vi "Parse.vi"(8 "Error In":errorcluster, 11 "Reader":refnum<class "Abstract.lvclass">) -> (0 "Error Out":errorcluster, 3 "Tokens":refnum<class "Abstract.lvclass">[](array[class]))   [LabVIEW 2018, in "Toolkit.lvlib" / "Parser.lvclass"]
uses:
  Parser.lvclass
  Tokens/Abstract/Abstract.lvclass
  Readers/Abstract/Abstract.lvclass
  Parser.lvclass/Parser.ctl
  Support/Is Open Delimiter.vi
  Support/Pop Content.vi
  Support/Has Content.vi
  Support/Add Text Token.vi
  Support/Peek Content.vi
  Support/Is Close Delimiter.vi
  Support/Tokenize Tag.vi
  Support/Ignore Comment.vi
  Support/Change Delimiters.vi
  Tokens/Text/Text.lvclass
  D:/Users/cfield/Code/Field R&D Services/Mustache/trunk/src/Toolkit/Tokens/Abstract/Abstract.lvclass
  Tokens/EscapedVariable/EscapedVariable.lvclass
  D:/Users/cfield/Code/Field R&D Services/Mustache/trunk/src/Toolkit/Tokens/Keyable/API/Keyable.lvclass
  Tokens/UnescapedVariable/UnescapedVariable.lvclass
  Tokens/BeginSection/BeginSection.lvclass
  Tokens/InvertedSection/InvertedSection.lvclass
  Tokens/EndSection/EndSection.lvclass
  Tokens/Partial/Partial.lvclass
  Tokens/Keyable/API/Keyable.lvclass
  Tokens/Text/API/New.vi
  <vilib>/Utility/error.llb/Trim Whitespace.vi
  Tokens/EscapedVariable/API/New.vi
  Tokens/UnescapedVariable/API/New.vi
  Tokens/BeginSection/API/New.vi
  Tokens/InvertedSection/API/New.vi
  Tokens/EndSection/API/New.vi
  Tokens/Partial/API/New.vi
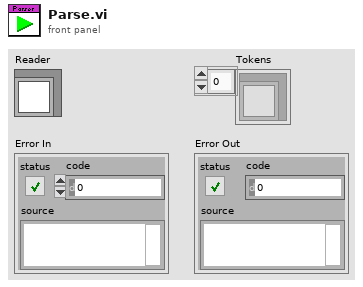
[diagram p1: front panel]
types:
  T1 = typedef "Toolkit.lvlib/Parser.lvclass/States.ctl" = enum16{"Text", "Open Delimiter", "Tag Type", "Tag Key", "Close Delimiter"}
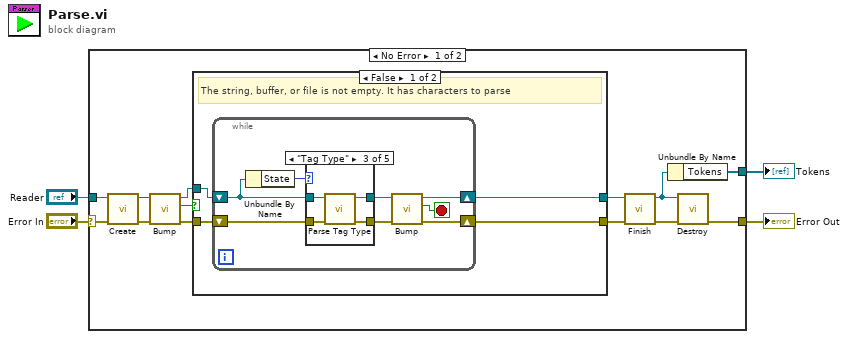
[diagram p0: block diagram]
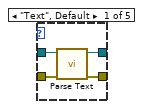
[diagram p2: hidden frame]
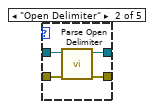
[diagram p3: hidden frame]
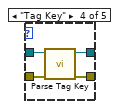
[diagram p4: hidden frame]
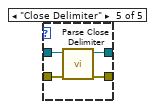
[diagram p5: hidden frame]
diagram:
  n1 = case shown="No Error" "Error In" {
    selector: "Error In" -> [w10 w52]
    tunnel: "Reader" -> [w11 _]
    tunnel: [w5 w52] -> w3
    tunnel: [w16 _] -> w2
    frame No Error {
      n2 = call "Create.vi"("Error In"=w10, "Reader"=w11) -> ("Error Out"=w9:errorcluster, "Parser"=w8:refnum<class "Parser.lvclass">)  [unwired: 8 in]
      n3 = call "Bump.vi"("Error In"=w9, "Parser In"=w8) -> ("Error Out"=w14:errorcluster, "Done"=w13:bool, "Parser Out"=w15:refnum<class "Parser.lvclass">)  [unwired: 7 in]
      n4 = case shown="False" w13 {
        tunnel: [w19 w50] -> w12
        tunnel: [w18 w51] -> w17
        tunnel: w14 -> [w21 w50]
        tunnel: w15 -> [w20 w51]
        frame False {
          # "The string, buffer, or file is not empty. It has characters to parse"
          n5 = while {
            shift-right: [w23] -> w19
            shift-left: w21 -> [w27]
            shift-right: [w25] -> w18
            shift-left: w20 -> [w28]
            stop <- w24 stop-if-true
            n6 = Unbundle By Name(w28) -> ("State"=w29:T1)
            n7 = case shown="\"Tag Type\"" w29 {
              tunnel: w27 -> [w32 w37 w38 w42 w46]
              tunnel: w28 -> [w33 w36 w41 w45 w49]
              tunnel: [w31 w35 w40 w44 w48] -> w26
              tunnel: [w30 w34 w39 w43 w47] -> w22
              frame "Text", Default {
                n8 = call "Parse Text.vi"("Error In"=w32, "Parser In"=w33) -> ("Error Out"=w30:errorcluster, "Parser Out"=w31:refnum<class "Parser.lvclass">)  [unwired: 8 in]
              }
              frame "Open Delimiter" {
                n9 = call "Parse Open Delimiter.vi"("Error In"=w37, "Parser In"=w36) -> ("Error Out"=w34:errorcluster, "Parser Out"=w35:refnum<class "Parser.lvclass">)  [unwired: 8 in]
              }
              frame "Tag Type" {
                n10 = call "Parse Tag Type.vi"("Error In"=w38, "Parser In"=w41) -> ("Error Out"=w39:errorcluster, "Parser Out"=w40:refnum<class "Parser.lvclass">)  [unwired: 8 in]
              }
              frame "Tag Key" {
                n11 = call "Parse Tag Key.vi"("Error In"=w42, "Parser In"=w45) -> ("Error Out"=w43:errorcluster, "Parser Out"=w44:refnum<class "Parser.lvclass">)  [unwired: 8 in]
              }
              frame "Close Delimiter" {
                n12 = call "Parse Close Delimiter.vi"("Error In"=w46, "Parser In"=w49) -> ("Error Out"=w47:errorcluster, "Parser Out"=w48:refnum<class "Parser.lvclass">)  [unwired: 8 in]
              }
            }
            n13 = call "Bump.vi"("Error In"=w22, "Parser In"=w26) -> ("Error Out"=w23:errorcluster, "Done"=w24:bool, "Parser Out"=w25:refnum<class "Parser.lvclass">)  [unwired: 7 in]
          }
        }
        frame True {
          # "The string, buffer, file, etc. is empty. There is nothing to do."
        }
      }
      n14 = call "Finish.vi"("Error In"=w12, "Parser In"=w17) -> ("Error Out"=w6:errorcluster, "Parser Out"=w7:refnum<class "Parser.lvclass">)  [unwired: 8 in]
      n15 = Unbundle By Name(w7) -> ("Tokens"=w16:refnum<class "Abstract.lvclass">[])
      n16 = call "Destroy.vi"("Error In"=w6, "Parser"=w7) -> ("Error Out"=w5:errorcluster)  [unwired: 9 in]
    }
    frame Error {
    }
  }
  "Error Out" <- w3
  "Tokens" <- w2
